vi "Channel ID to Tree Items.vi"(8 "error in (no error)":errorcluster, 9 "Channel ID":string, 11 "Application Data in":T2) -> (0 "error out":errorcluster, 1 "Settings":T1, 2 "Item":T1, 3 "Application Data out":T2)   [LabVIEW 2017, in "DSF Configuration Utility.lvlib"]
uses:
  DSF Configuration Utility.lvlib
  Main VI/Application Data.ctl
  DSF Configuration API/1.0.0/Public/Controls/DSF Config Data RefNum.ctl
  Main VI/Window State.ctl
  Main VI/View Mode.ctl
  Tree Item Management/Tree Item.ctl
  Tree Item Type.ctl
  DSF Configuration API/1.0.0/Public/Read Item/Read Channel.vi
  DSF Configuration API/1.0.0/Public/Read Item/Read Settings.vi
  DSF Configuration API/1.0.0/DSF Configuration API.lvlib
panel:
  # "App\nData"
  # "App\nData"
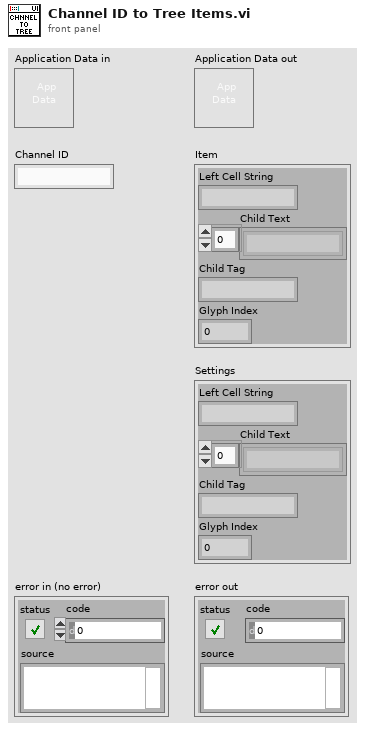
[diagram p1: front panel]
types:
  T1 = typedef "DSF Configuration Utility.lvlib/Tree Item.ctl" = cluster{"Left Cell String":string, "Child Text":string[], "Child Tag":string, "Glyph Index":i32}
  T2 = typedef "DSF Configuration Utility.lvlib/Application Data.ctl" = cluster{"DSF Refnum out":T3, "Tree Control":refnum<vi>, "Tab Control":refnum<vi>, "Top-Level VI":refnum<vi>, "value control refs":refnum<vi>[], "View State":T4}
  T3 = typedef "DSF Configuration API.lvlib/DSF Config Data RefNum.ctl" = refnum<k1>
  T4 = typedef "DSF Configuration Utility.lvlib/View Mode.ctl" = enum16{"Tree", "List"}
  T5 = typedef "DSF Configuration Utility.lvlib/Tree Item Type.ctl" = enum16{"Plugin", "Group", "Transfer", "Channel", "Setting"}
  T6 = typedef "DSF Configuration API.lvlib/DSF Channel Info.ctl" = cluster{"count":i32, "offset":i32, "data type":i32, "resource path":string, "settings id":string}
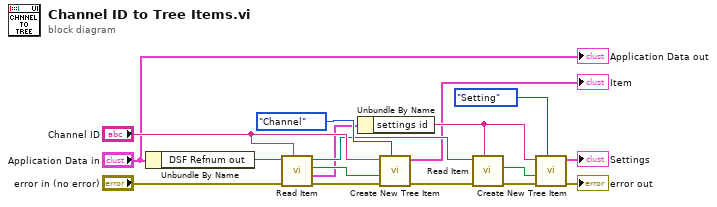
[diagram p0: block diagram]
diagram:
  n1 = Unbundle By Name("Application Data in") -> ("DSF Refnum out"=w4:T3)
  n2 = call-poly "Read Item.vi"("name"="Channel ID", "error in (no error)"="error in (no error)", "refnum"=w4) -> ("error out"=w12:errorcluster, "value"=w5:T6, "found?"=w9:bool, "refnum out"=w6:T3)  [unwired: 5 in]
  n3 = Unbundle By Name(w5) -> ("settings id"=w10:string)
  n4 = call "Create New Tree Item.vi"("Item Type"=Tree_Item_Type."Channel", "error in"=w12, "found?"=w9, "Left Cell String"="Channel ID") -> ("error out"=w13:errorcluster, "Item"=→"Item":T1)  [unwired: 6 in]
  n5 = call-poly "Read Item.vi"("name"=w10, "error in (no error)"=w13, "refnum"=w6) -> ("error out"=w14:errorcluster, "found?"=w11:bool)  [unwired: 5 in, 2 out]
  n6 = call "Create New Tree Item.vi"("Item Type"=Tree_Item_Type."Setting", "error in"=w14, "found?"=w11, "Left Cell String"=w10) -> ("error out"=→"error out":errorcluster, "Item"=→"Settings":T1)  [unwired: 6 in]
  "Application Data out" <- "Application Data in"
